vi "Ejemplo 3.vi"() -> ()   [LabVIEW 2020]
panel:
  in  "stop":bool
  out "cruce por cero":dbl
  out "pendiente (m)":dbl
  in  "y2":dbl
  in  "y1":dbl
  in  "x2":dbl
  in  "x1":dbl
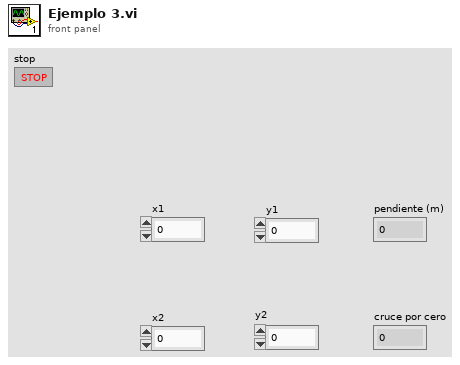
[diagram p1: front panel]
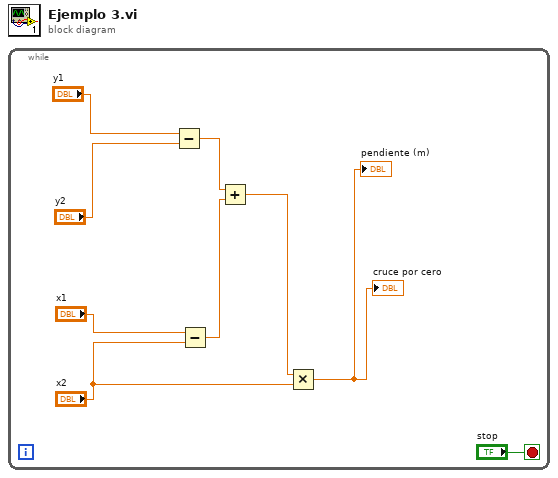
[diagram p0: block diagram]
diagram:
  n1 = while {
    stop <- "stop" stop-if-true
    n2 = Subtract(x="y1", y="y2") -> (x-y=w6:dbl)
    n3 = Subtract(x="x1", y="x2") -> (x-y=w5:dbl)
    n4 = Add(x=w6, y=w5) -> (x+y=w4:dbl)
    n5 = Multiply(x=w4, y="x2") -> (x*y=→"pendiente (m)" →"cruce por cero":dbl)
  }
